vi "Begin.vi"() -> (0 "error out":errorcluster)   [LabVIEW 2014]
doc: "Called before other user functions, this VI is expected to open initial I/O refnums, load in file data, and do all program initialization. Notice that the <B>error out</B> terminal is simply used for data flow. Wiring it to other structures or subVIs ensures that this VI runs first."
uses:
  <vilib>/Rock Robotics/WPI/DriverStation/WPI_DriverStationRobotMode2.ctl
  <vilib>/Rock Robotics/WPI/Relay/WPI_RelayDirection.ctl
  <vilib>/Rock Robotics/SystemInterfaces/Typedef/FPGA_TypedefDigitalModule.ctl
  <vilib>/Rock Robotics/WPI/SafetyOutput/WPI_SafetyOutputConfigMenu.ctl
  <vilib>/Rock Robotics/WPI/Joystick/WPI_JoystickDeviceEnum.ctl
  <vilib>/Rock Robotics/SystemInterfaces/DIO/FPGA_DIOChannel.ctl
  <vilib>/Rock Robotics/WPI/Encoder/WPI_EncoderType.ctl
  <vilib>/Rock Robotics/SystemInterfaces/AI/FPGA_AIGyroChannel.ctl
  <vilib>/Rock Robotics/SystemInterfaces/Typedef/FPGA_TypedefAnalogModuleForGyro.ctl
  <vilib>/Rock Robotics/SystemInterfaces/AI/FPGA_AIChannel.ctl
  <vilib>/Rock Robotics/SystemInterfaces/DIO/FPGA_DIORelayChannel.ctl
  <vilib>/Rock Robotics/WPI/CAN/Jaguar/SubVIs/WPI_CANJaguar_ControlMode.ctl
  Robot Global Data.vi
  <vilib>/Rock Robotics/WPI/RobotDrive/WPI_RobotDriveOpen4MotorWithCANJaguar.vi
  <vilib>/Rock Robotics/WPI/Counter/WPI_CounterDigitalInputToDigitalSource.vi
  <vilib>/Rock Robotics/WPI/Ultrasonic/WPI_SonarMB1010AnalogOpen.vi
  <vilib>/Rock Robotics/WPI/Ultrasonic/WPI_SonarMB1010AnalogRefNum Registry Set.vi
  <vilib>/Rock Robotics/WPI/MotorControl/WPI_MotorControlOpenCANJaguar.vi
  <vilib>/Rock Robotics/WPI/Camera/WPI_CameraFrameRate.ctl
  <vilib>/Rock Robotics/WPI/Camera/WPI_CameraWhite Balance Values.ctl
  <vilib>/Rock Robotics/WPI/Camera/WPI_CameraExposure Values.ctl
  <vilib>/Rock Robotics/WPI/Camera/WPI_CameraImageSize.ctl
  <vilib>/Rock Robotics/WPI/Camera/WPI_CameraExposure Priority Values.ctl
  <vilib>/Rock Robotics/SystemInterfaces/Typedef/FPGA_TypedefAnalogModule.ctl
panel:
  # "Launch Angle Position PID"
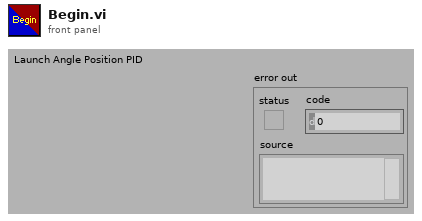
[diagram p1: front panel]
types:
  T1 = typedef "WPI_SafetyOutputConfigMenu.ctl" = enum16{"Enable", "Disable"}
  T2 = typedef "FPGA_TypedefDigitalModule.ctl" = enum16{"Controller 1"}
  T3 = typedef "WPI_RelayDirection.ctl" = enum16{"Both directions", "Forward only", "Reverse only"}
  T4 = typedef "WPI_DriverStationRobotMode2.ctl" = enum16{"Autonomous Disabled", "Autonomous Enabled", "Teleop Disabled", "Teleop Enabled", "Disconnected", "Finish", "Test Disabled", "Test Enabled"}
  T5 = typedef "WPI_JoystickDeviceEnum.ctl" = enum16{"USB 0", "USB 1", "USB 2", "USB 3", "USB 4", "USB 5"}
  T6 = typedef "WPI_CameraExposure Priority Values.ctl" = enum16{"None", "Prioritize frame rate", "Prioritize image quality"}
  T7 = typedef "WPI_CameraImageSize.ctl" = enum16{"640x480", "320x240", "160x120", "Custom"}
  T8 = typedef "WPI_CameraExposure Values.ctl" = enum16{"Auto", "Flicker-free 50 Hz", "Flicker-free 60 Hz", "Hold current", "Custom"}
  T9 = typedef "WPI_CameraWhite Balance Values.ctl" = enum16{"Auto", "Fixed indoor", "Fixed outdoor 1", "Fixed outdoor 2", "Fixed fluorescent 1", "Fixed fluorescent 2", "Hold current", "Custom"}
  T10 = typedef "WPI_CameraFrameRate.ctl" = u32
  T11 = typedef "FPGA_DIOChannel.ctl" = enum8{"DIO 0", "DIO 1", "DIO 2", "DIO 3", "DIO 4", "DIO 5", "DIO 6", "DIO 7", "DIO 8", "DIO 9", "DIO MXP 0", "DIO MXP 1", "DIO MXP 2", "DIO MXP 3", "DIO MXP 4", "DIO MXP 5", "DIO MXP 6", "DIO MXP 7", "DIO MXP 8", "DIO MXP 9", "DIO MXP 10", "DIO MXP 11", "DIO MXP 12", "DIO MXP 13", "DIO MXP 14", "DIO MXP 15", "Invalid"}
  T12 = typedef "FPGA_TypedefAnalogModuleForGyro.ctl" = enum16{"Controller 1"}
  T13 = typedef "FPGA_AIGyroChannel.ctl" = enum8{"AI 0", "AI 1", "Invalid"}
  T14 = typedef "FPGA_TypedefAnalogModule.ctl" = enum16{"Controller 1"}
  T15 = typedef "FPGA_AIChannel.ctl" = enum8{"AI 0", "AI 1", "AI 2", "AI 3", "AI MXP 0", "AI MXP 1", "AI MXP 2", "AI MXP 3", "Invalid"}
  T16 = typedef "FPGA_DIORelayChannel.ctl" = enum8{"Relay 0", "Relay 1", "Relay 2", "Relay 3", "Invalid"}
  T17 = typedef "WPI_CANJaguar_ControlMode.ctl" = enum8{"Percent VBus", "Current", "Speed", "Position", "Voltage"}
  T18 = typedef "WPI_JoystickDevRef.ctl" = cluster{"Device":T5}
  T19 = typedef "WPI_CameraDevRef.ctl" = cluster{"Camera Address":string, "CameraStatus":errorcluster}
  T20 = typedef "WPI_RobotDriveDevRef.ctl" = cluster{"DevStatus":errorcluster, "Motors[]":T21[], "Square Inputs":bool, "Max Output":dbl}
  T21 = typedef "WPI_MotorControlDeviceRef.ctl" = cluster{"DeviceStatus":errorcluster, "Type":enum16{"PWM", "CAN"}, "PWM":cluster{"Controller":T2, "PWM Channel":T22, "DeadBand":T23}, "CAN":cluster{"Device Number":u8, "Control Mode":T17, "Semaphore":T24, "Max Vout":dbl}, "Invert":bool, "TransformRef":T25, "InvTransformRef":T25}
  T22 = typedef "FPGA_DIOPWMChannel.ctl" = enum8{"PWM 0", "PWM 1", "PWM 2", "PWM 3", "PWM 4", "PWM 5", "PWM 6", "PWM 7", "PWM 8", "PWM 9", "PWM MXP 0", "PWM MXP 1", "PWM MXP 2", "PWM MXP 3", "PWM MXP 4", "PWM MXP 5", "PWM MXP 6", "PWM MXP 7", "PWM MXP 8", "PWM MXP 9", "Invalid"}
  T23 = typedef "WPI_PWMDeadband.ctl" = cluster{"Name":string, "maxPositivePwm":i32, "minPositivePwm":i32, "centerPwm":i32, "maxNegativePwm":i32, "minNegativePwm":i32, "angularRange":u16}
  T24 = typedef "Semaphore RefNum" = refnum<k1>
  T25 = typedef "WPI_PWMTransform_ConPane.ctl" = refnum<vi>
  T26 = typedef "WPI_EncoderType.ctl" = enum16{"1x", "2x", "4x"}
  T27 = typedef "WPI_DigitalInputDevRef.ctl" = cluster{"DevStatus":errorcluster, "DIO Channel":T11, "Controller":T2}
  T28 = typedef "FPGA_CounterEncoderSourceConvertionLVSourceType.ctl" = cluster{"DevStatus":errorcluster, "AnalogTriggerMode?":bool, "DigitalMode":cluster{"Controller":T2, "DIO Channel":T29}, "AnalogTriggerMode":cluster{"AnalogTriggerIndex":T30, "OutputType":T31}}
  T29 = typedef "FPGA_DIODigitalSourceChannel.ctl" = enum8{"DIO 0", "DIO 1", "DIO 2", "DIO 3", "DIO 4", "DIO 5", "DIO 6", "DIO 7", "DIO 8", "DIO 9", "DIO MXP 0", "DIO MXP 1", "DIO MXP 2", "DIO MXP 3", "DIO MXP 4", "DIO MXP 5", "DIO MXP 6", "DIO MXP 7", "DIO MXP 8", "DIO MXP 9", "DIO MXP 10", "DIO MXP 11", "DIO MXP 12", "DIO MXP 13", "DIO MXP 14", "DIO MXP 15", "Disabled"}
  T30 = typedef "FPGA_AnalogTriggerIndex.ctl" = enum8{"Trig 0", "Trig 1", "Trig 2", "Trig 3", "Trig 4", "Trig 5", "Trig 6", "Trig 7", "Invalid"}
  T31 = typedef "FPGA_AnalogTriggerOutType.ctl" = enum16{"InWindow", "TriggerState", "Rising", "Falling"}
  T32 = typedef "WPI_EncoderDevRef.ctl" = cluster{"DevStatus":errorcluster, "EncoderIndex":T33, "CounterIndex":T34, "DistancePerCount":dbl, "Decoding Type":T26}
  T33 = typedef "FPGA_EncoderIdx.ctl" = enum8{"Enc 0", "Enc 1", "Enc 2", "Enc 3", "Invalid"}
  T34 = typedef "FPGA_CounterCtrSystemIndex.ctl" = enum8{"Ctr 0", "Ctr 1", "Ctr 2", "Ctr 3", "Ctr 4", "Ctr 5", "Ctr 6", "Ctr 7", "Invalid"}
  T35 = typedef "WPI_GyroDevRef.ctl" = cluster{"DevStatus":errorcluster, "Analog Module":T14, "Analog Channel":T15, "Offset":dbl, "Gain (VoltsPerDegree/Second)":dbl}
  T36 = typedef "WPI_AnalogChannelDevRef.ctl" = cluster{"DevStatus":errorcluster, "Controller":T14, "Analog Channel":T15}
  T37 = typedef "WPI_SonarMB1010AnalogDeviceRef.ctl" = cluster{"AIDeviceRef":T36, "Scaling factor (V/in)":dbl, "Average Bits":u8}
  T38 = typedef "WPI_RelayDevRef.ctl" = cluster{"DevStatus":errorcluster, "Relay Channel":T16, "Controller":T2, "Relay Direction":T3}
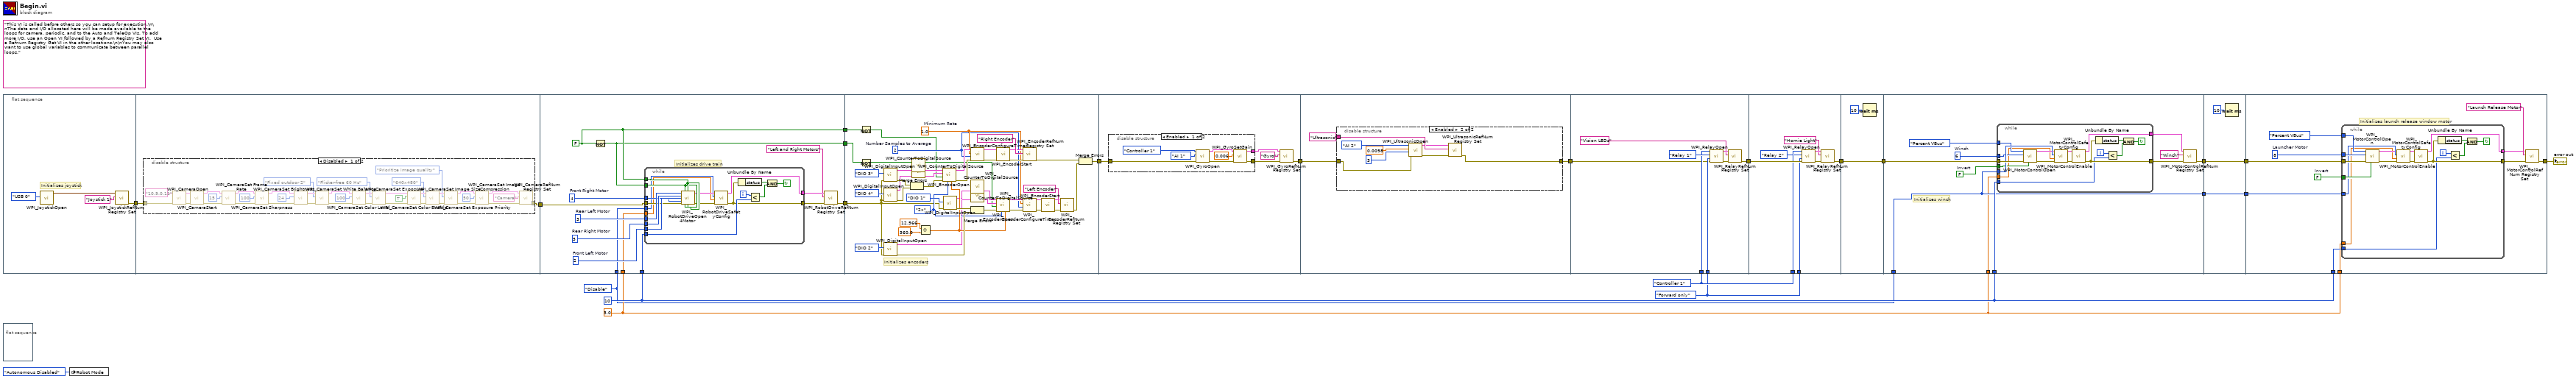
[diagram p0: block diagram]
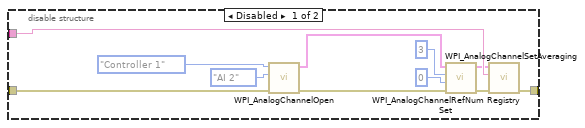
[diagram p4: hidden frame]
diagram:
  w10 = WPI_SafetyOutputConfigMenu."Disable" ("mode")
  w11 = 3.0 ("timeout (s)")
  w7 = FPGA_TypedefDigitalModule."Controller 1" ("Digital Module (Module 1)")
  w6 = WPI_RelayDirection."Forward only" ("Relay Direction")
  w13 = 10 ("y")
  (unwired) "This VI is called before others so you can setup for execution.\n\nThe data and I/O allocated here will be made available to the loops for camera, periodic, and to the Auto and TeleOp VIs. To add more I/O, use an Open VI followed by a Refnum Registry Set VI.  Use a Refnum Registry Get VI in the other locations.\n\nYou may also want to use global variables to communicate between parallel loops."
  n1 = flat-sequence {
    tunnel: [w23] -> w5
    tunnel: w5 -> [w28]
    tunnel: [w27] -> w1
    tunnel: [w73] -> w22
    tunnel: [w72] -> w21
    tunnel: [w71] -> w20
    tunnel: w13 -> [w70]
    tunnel: w11 -> [w69]
    tunnel: w10 -> [w68]
    tunnel: w1 -> [w67]
    tunnel: w20 -> [w104]
    tunnel: w21 -> [w103]
    tunnel: w22 -> [w102]
    tunnel: [w99] -> w12
    tunnel: [w145] -> w8
    tunnel: w12 -> [w149]
    tunnel: w8 -> [w160]
    tunnel: [w158] -> w2
    tunnel: w6 -> [w183]
    tunnel: w7 -> [w182]
    tunnel: [w181] -> w9
    tunnel: w2 -> [w180]
    tunnel: w9 -> [w192]
    tunnel: w6 -> [w191]
    tunnel: w7 -> [w190]
    tunnel: [w188] -> w4
    tunnel: [w196] -> w14
    tunnel: w4 -> [w196]
    tunnel: [w207] -> w18
    tunnel: [w199] -> w16
    tunnel: w13 -> [w204]
    tunnel: w14 -> [w200]
    tunnel: w10 -> [w199]
    tunnel: w11 -> [w198]
    tunnel: w18 -> [w228]
    tunnel: [w228] -> w17
    tunnel: w16 -> [w227]
    tunnel: [w227] -> w15
    tunnel: w17 -> [w235]
    tunnel: w15 -> [w234]
    tunnel: w13 -> [w231]
    tunnel: w11 -> [w230]
    tunnel: [w229] -> w3
    frame #0 {
      # "Initializes joystick"
      n2 = call <vilib>:"WPI_JoystickOpen.vi"("JoystickDevice"=WPI_JoystickDeviceEnum."USB 0") -> ("JoystickDevRef"=w25:T18)  [unwired: 10 in]
      n3 = call <vilib>:"WPI_JoystickRefNum Registry Set.vi"("refnum name"="Joystick 1", "JoystickDevRef"=w25) -> ("error out"=w23:errorcluster)  [unwired: 8 in, 1 out]
    }
    frame #1 {
      n4 = disable-structure shown="Disabled" {
        disable-tunnel: w28 -> [w66 _]
        disable-tunnel: [w29 _] -> w27
        frame Disabled {
          n5 = call <vilib>:"WPI_CameraOpen.vi"("error in (no error)"=w66, "Camera Address"="10.9.0.11") -> ("error out"=w65:errorcluster, "CameraDevRef"=w63:T19)  [unwired: 8 in]
          n6 = call <vilib>:"WPI_CameraStart.vi"("error in (no error)"=w65, "CameraDevRef"=w63) -> ("error out"=w60:errorcluster, "CameraDevRef Out"=w61:T19)  [unwired: 8 in]
          n7 = call <vilib>:"WPI_CameraSet Frame Rate.vi"("error in (no error)"=w60, "Frame Rate (fps)"=T10 15, "CameraDevRef"=w61) -> ("error out"=w58:errorcluster, "CameraDevRef Out"=w59:T19)  [unwired: 7 in]
          n8 = call <vilib>:"WPI_CameraSet Sharpness.vi"("error in (no error)"=w58, "Sharpness"=100, "CameraDevRef"=w59) -> ("error out"=w56:errorcluster, "CameraDevRef Out"=w57:T19)  [unwired: 7 in]
          n9 = call <vilib>:"WPI_CameraSet Brightness.vi"("error in (no error)"=w56, "Brightness"=24, "CameraDevRef"=w57) -> ("error out"=w54:errorcluster, "CameraDevRef Out"=w55:T19)  [unwired: 7 in]
          n10 = call <vilib>:"WPI_CameraSet White Balance.vi"("error in (no error)"=w54, "White Balance"=WPI_CameraWhite_Balance_Values."Fixed outdoor 2", "CameraDevRef"=w55) -> ("error out"=w52:errorcluster, "CameraDevRef Out"=w53:T19)  [unwired: 7 in]
          n11 = call <vilib>:"WPI_CameraSet Color Level.vi"("error in (no error)"=w52, "Color Level"=100, "CameraDevRef"=w53) -> ("error out"=w51:errorcluster, "CameraDevRef Out"=w50:T19)  [unwired: 7 in]
          n12 = call <vilib>:"WPI_CameraSet Exposure.vi"("error in (no error)"=w51, "Exposure"=WPI_CameraExposure_Values."Flicker-free 60 Hz", "CameraDevRef"=w50) -> ("error out"=w49:errorcluster, "CameraDevRef Out"=w48:T19)  [unwired: 7 in]
          n13 = call <vilib>:"WPI_CameraSet Color Enable.vi"("error in (no error)"=w49, "Color Enabled"=TRUE, "CameraDevRef"=w48) -> ("error out"=w46:errorcluster, "CameraDevRef Out"=w47:T19)  [unwired: 7 in]
          n14 = call <vilib>:"WPI_CameraSet Image Size.vi"("error in (no error)"=w46, "Image Size"=WPI_CameraImageSize."640x480", "CameraDevRef"=w47) -> ("error out"=w44:errorcluster, "CameraDevRef Out"=w45:T19)  [unwired: 7 in]
          n15 = call <vilib>:"WPI_CameraSet Exposure Priority.vi"("error in (no error)"=w44, "Exposure Priority"=WPI_CameraExposure_Priority_Values."Prioritize image quality", "CameraDevRef"=w45) -> ("error out"=w43:errorcluster, "CameraDevRef Out"=w42:T19)  [unwired: 7 in]
          n16 = call <vilib>:"WPI_CameraSet Image Compression.vi"("error in (no error)"=w43, "Compression"=50, "CameraDevRef"=w42) -> ("error out"=w40:errorcluster, "CameraDevRef Out"=w41:T19)  [unwired: 7 in]
          n17 = call <vilib>:"WPI_CameraRefNum Registry Set.vi"("error in (no error)"=w40, "refnum name"="Camera", "CameraDevRef"=w41) -> ("error out"=w29:errorcluster)  [unwired: 7 in, 1 out]
        }
        frame Enabled {
        }
      }
    }
    frame #2 {
      w72 = FALSE ("Rear Left Motor Inverted")
      w74 = u8 4  # Front Right Motor
      w75 = u8 2  # Front Left Motor
      w76 = u8 5  # Rear Right Motor
      w77 = u8 3  # Rear Left Motor
      # "Initializes drive train"
      n18 = Not(x=w72) -> (.not. x?=w71:bool)
      n19 = while {
        tunnel: [w85] -> w80
        tunnel: [w86] -> w79
        tunnel: w77 -> [w98]
        tunnel: w76 -> [w97]
        tunnel: w75 -> [w96]
        tunnel: w74 -> [w95]
        tunnel: w67 -> [w94]
        tunnel: w72 -> [w93]
        tunnel: w71 -> [w92]
        tunnel: w70 -> [w88]
        tunnel: w68 -> [w82]
        tunnel: w69 -> [w81]
        i -> [w89]
        stop <- w91 continue-if-true
        n20 = call-poly <vilib>:"WPI_RobotDriveOpen4Motor.vi"("Rear Left Motor"=w98, "Rear Left Motor Inverted"=w92, "Rear Right Motor Inverted"=w93, "Rear Right Motor"=w97, "Front Left Motor"=w96, "Front Right Motor"=w95, "error in (no error)"=w94, "Front Left Motor Inverted"=w92, "Front Right Motor Inverted"=w93) -> ("RobotDriveDevRef"=w84:T20, "error out"=w83:errorcluster)  [unwired: 5 in]
        n21 = call <vilib>:"WPI_RobotDriveSafetyConfig.vi"("error in (no error)"=w83, "timeout (s)"=w81, "mode"=w82, "RobotDriveDevRef"=w84) -> ("error out"=w85:errorcluster, "RobotDriveDevRef"=w86:T20)  [unwired: 6 in]
        n22 = Unbundle By Name(w85) -> ("status"=w90:bool)
        n23 = Less?(x=w89, y=w88) -> (x < y?=w87:bool)
        n24 = And(x=w90, y=w87) -> (x .and. y?=w91:bool)
      }
      n25 = call <vilib>:"WPI_RobotDriveRefNum Registry Set.vi"("error in (no error)"=w80, "refnum name"="Left and Right Motors", "RobotDriveDevRef"=w79) -> ("error out"=w73:errorcluster)  [unwired: 7 in, 1 out]
    }
    frame #3 {
      w112 = u8 2  # Number Samples to Average
      w113 = 1.0  # Minimum Rate
      w122 = WPI_EncoderType."2x" ("Decoding Type")
      # "Initializes encoders"
      n26 = Not(x=w103) -> (.not. x?=w106:bool)
      n27 = Not(x=w104) -> (.not. x?=w107:bool)
      n28 = call <vilib>:"WPI_DigitalInputOpen.vi"("error in (no error)"=w102, "DIO Channel"=FPGA_DIOChannel."DIO 3") -> ("error out"=w143:errorcluster, "DigitalInputDevRef"=w111:T27)  [unwired: 8 in]
      n29 = call <vilib>:"WPI_DigitalInputOpen.vi"("error in (no error)"=w102, "DIO Channel"=FPGA_DIOChannel."DIO 4") -> ("error out"=w142:errorcluster, "DigitalInputDevRef"=w110:T27)  [unwired: 8 in]
      n30 = call <vilib>:"WPI_DigitalInputOpen.vi"("error in (no error)"=w102, "DIO Channel"=FPGA_DIOChannel."DIO 2") -> ("error out"=w137:errorcluster, "DigitalInputDevRef"=w109:T27)  [unwired: 8 in]
      n31 = Merge Errors(w143, w142) -> (w141:errorcluster)
      n32 = call-poly <vilib>:"WPI_CounterToDigitalSource.vi"("DigitalInputDevRef"=w111) -> ("Digital Source"=w144:T28)  [unwired: 6 in]
      n33 = call-poly <vilib>:"WPI_CounterToDigitalSource.vi"("DigitalInputDevRef"=w110) -> ("Digital Source"=w140:T28)  [unwired: 6 in]
      n34 = Divide(x=12.566, y=360.0) -> (x/y=w127:dbl)
      n35 = call <vilib>:"WPI_EncoderOpen.vi"("DistancePerCount"=w127, "Decoding Type"=w122, "error in (no error)"=w141, "Invert Direction (False)"=w106, "BSource"=w140, "ASource"=w144) -> ("error out"=w114:errorcluster, "EncoderDevRef"=w117:T32)  [unwired: 4 in]
      n36 = call <vilib>:"WPI_DigitalInputOpen.vi"("error in (no error)"=w102, "DIO Channel"=FPGA_DIOChannel."DIO 1") -> ("error out"=w138:errorcluster, "DigitalInputDevRef"=w108:T27)  [unwired: 8 in]
      n37 = call <vilib>:"WPI_EncoderConfigureTimer.vi"("error in (no error)"=w114, "Number Samples to Average"=w112, "Minimum Rate"=w113, "EncoderDevRef"=w117) -> ("error out"=w115:errorcluster, "EncoderDevRef"=w116:T32)  [unwired: 6 in]
      n38 = call-poly <vilib>:"WPI_CounterToDigitalSource.vi"("DigitalInputDevRef"=w108) -> ("Digital Source"=w139:T28)  [unwired: 6 in]
      n39 = call-poly <vilib>:"WPI_CounterToDigitalSource.vi"("DigitalInputDevRef"=w109) -> ("Digital Source"=w135:T28)  [unwired: 6 in]
      n40 = Merge Errors(w138, w137) -> (w136:errorcluster)
      n41 = call <vilib>:"WPI_EncoderOpen.vi"("DistancePerCount"=w127, "Decoding Type"=w122, "error in (no error)"=w136, "Invert Direction (False)"=w107, "BSource"=w135, "ASource"=w139) -> ("error out"=w120:errorcluster, "EncoderDevRef"=w121:T32)  [unwired: 4 in]
      n42 = call <vilib>:"WPI_EncoderStart.vi"("error in (no error)"=w115, "EncoderDevRef"=w116) -> ("error out"=w123:errorcluster, "EncoderDevRef"=w124:T32)  [unwired: 8 in]
      n43 = call <vilib>:"WPI_EncoderRefNum Registry Set.vi"("error in (no error)"=w123, "refnum name"="Right Encoder", "EncoderDevRef"=w124) -> ("error out"=w101:errorcluster)  [unwired: 7 in, 1 out]
      n44 = call <vilib>:"WPI_EncoderConfigureTimer.vi"("error in (no error)"=w120, "Number Samples to Average"=w112, "Minimum Rate"=w113, "EncoderDevRef"=w121) -> ("error out"=w118:errorcluster, "EncoderDevRef"=w119:T32)  [unwired: 6 in]
      n45 = call <vilib>:"WPI_EncoderStart.vi"("error in (no error)"=w118, "EncoderDevRef"=w119) -> ("error out"=w125:errorcluster, "EncoderDevRef"=w126:T32)  [unwired: 8 in]
      n46 = call <vilib>:"WPI_EncoderRefNum Registry Set.vi"("error in (no error)"=w125, "refnum name"="Left Encoder", "EncoderDevRef"=w126) -> ("error out"=w100:errorcluster)  [unwired: 7 in, 1 out]
      n47 = Merge Errors(w101, w100) -> (w99:errorcluster)
    }
    frame #4 {
      n48 = disable-structure shown="Enabled" {
        disable-tunnel: w149 -> [w157 _]
        disable-tunnel: [w151 _] -> w146
        disable-tunnel: [w150 _] -> w148
        frame Enabled {
          n49 = call <vilib>:"WPI_GyroOpen.vi"("error in (no error)"=w157, "Analog Channel"=FPGA_AIGyroChannel."AI 1", "Controller"=FPGA_TypedefAnalogModuleForGyro."Controller 1" ("Analog Module (Module 1)")) -> ("error out"=w154:errorcluster, "GyroDevRef"=w153:T35)  [unwired: 6 in, 1 out]
          n50 = call <vilib>:"WPI_GyroSetGain.vi"("error in (no error)"=w154, "Gain (VoltsPerDegree/Second)"=0.006, "GyroDevRef"=w153) -> ("error out"=w150:errorcluster, "GyroDevRef"=w151:T35)  [unwired: 7 in]
        }
        frame Disabled {
        }
      }
      n51 = call <vilib>:"WPI_GyroRefNum Registry Set.vi"("error in (no error)"=w148, "refnum name"="Gyro", "GyroDevRef"=w146) -> ("error out"=w145:errorcluster)  [unwired: 7 in, 1 out]
    }
    frame #5 {
      n52 = disable-structure shown="Enabled" {
        disable-tunnel: w160 -> [w171 w179]
        disable-tunnel: [w164 w175] -> w158
        disable-tunnel: "Ultrasonic" ("refnum name") -> [w166 w173]
        frame Disabled {
          n53 = call <vilib>:"WPI_AnalogChannelOpen.vi"("error in (no error)"=w171, "Analog Channel"=FPGA_AIChannel."AI 2", "Controller"=FPGA_TypedefAnalogModule."Controller 1" ("Analog Module (Module 1)")) -> ("error out"=w161:errorcluster, "AIDeviceRef"=w170:T36)  [unwired: 7 in]
          n54 = call <vilib>:"WPI_AnalogChannelSetAveraging.vi"("error in (no error)"=w161, "OversampleBits"=u8 0, "AverageBits"=u8 3, "AIDeviceRef"=w170) -> ("error out"=w163:errorcluster, "AIDeviceRef"=w165:T36)  [unwired: 6 in]
          n55 = call <vilib>:"WPI_AnalogChannelRefNum Registry Set.vi"("error in (no error)"=w163, "refnum name"=w166, "AIDeviceRef"=w165) -> ("error out"=w164:errorcluster)  [unwired: 7 in, 1 out]
        }
        frame Enabled {
          n56 = call-poly <vilib>:"WPI_UltrasonicOpen.vi"("error in"=w179, "Average Bits"=u8 3, "Scaling factor (V/in)"=0.0098, "Analog Channel"=FPGA_AIChannel."AI 2") -> ("error out"=w174:errorcluster, "SonarMB1010AnalogDevRef"=w172:T37)  [unwired: 6 in]
          n57 = call-poly <vilib>:"WPI_UltrasonicRefNum Registry Set.vi"("error in (no error)"=w174, "refnum name"=w173, "SonarMB1010AnalogDevRef"=w172) -> ("error out"=w175:errorcluster)  [unwired: 7 in, 1 out]
        }
      }
    }
    frame #6 {
      n58 = call <vilib>:"WPI_RelayOpen.vi"("error in (no error)"=w180, "Relay Direction"=w183, "Relay Channel"=FPGA_DIORelayChannel."Relay 1", "Controller"=w182) -> ("error out"=w187:errorcluster, "RelayDevRef"=w186:T38)  [unwired: 6 in]
      n59 = call <vilib>:"WPI_RelayRefNum Registry Set.vi"("error in (no error)"=w187, "refnum name"="Vision LEDs", "RelayDevRef"=w186) -> ("error out"=w181:errorcluster)  [unwired: 7 in, 1 out]
    }
    frame #7 {
      n60 = call <vilib>:"WPI_RelayOpen.vi"("error in (no error)"=w192, "Relay Direction"=w191, "Relay Channel"=FPGA_DIORelayChannel."Relay 2", "Controller"=w190) -> ("error out"=w195:errorcluster, "RelayDevRef"=w194:T38)  [unwired: 6 in]
      n61 = call <vilib>:"WPI_RelayRefNum Registry Set.vi"("error in (no error)"=w195, "refnum name"="Homie Light", "RelayDevRef"=w194) -> ("error out"=w188:errorcluster)  [unwired: 7 in, 1 out]
    }
    frame #8 {
      n62 = Wait (ms)(milliseconds to wait=u32 10) -> ()  [unwired: 1 out]
    }
    frame #9 {
      w201 = FALSE  # Invert
      w202 = u8 6  # Winch
      # "Initializes winch"
      n63 = while {
        tunnel: w200 -> [w223]
        tunnel: w199 -> [w222]
        tunnel: [w218] -> w206
        tunnel: [w219] -> w205
        tunnel: w204 -> [w216]
        tunnel: WPI_CANJaguar_ControlMode."Percent VBus" ("Control Mode") -> [w212]
        tunnel: w202 -> [w211]
        tunnel: w201 -> [w210]
        tunnel: w198 -> [w209]
        i -> [w217]
        stop <- w213 continue-if-true
        n64 = call-poly <vilib>:"WPI_MotorControlOpen.vi"("Invert"=w210, "error in (no error)"=w223, "Device Number"=w211, "Control Mode"=w212) -> ("error out"=w220:errorcluster, "MotorControlDeviceRef"=w221:T21)  [unwired: 6 in]
        n65 = call <vilib>:"WPI_MotorControlSafetyConfig.vi"("error in (no error)"=w220, "timeout (s)"=w209, "mode"=w222, "MotorControlDevRef"=w221) -> ("error out"=w225:errorcluster, "MotorControlDevRef"=w224:T21)  [unwired: 6 in]
        n66 = call <vilib>:"WPI_MotorControlEnable.vi"("error in (no error)"=w225, "CAN Jaguar Ref"=w224) -> ("error out"=w218:errorcluster, "CAN Jaguar Ref Out"=w219:T21)  [unwired: 8 in]
        n67 = Unbundle By Name(w218) -> ("status"=w214:bool)
        n68 = Less?(x=w217, y=w216) -> (x < y?=w215:bool)
        n69 = And(x=w214, y=w215) -> (x .and. y?=w213:bool)
      }
      n70 = call <vilib>:"WPI_MotorControlRefNum Registry Set.vi"("error in (no error)"=w206, "refnum name"="Winch", "MotorControlDevRef"=w205) -> ("error out"=w207:errorcluster)  [unwired: 7 in, 1 out]
    }
    frame #10 {
      n71 = Wait (ms)(milliseconds to wait=u32 10) -> ()  [unwired: 1 out]
    }
    frame #11 {
      w238 = u8 8  # Launcher Motor
      w239 = FALSE  # Invert
      # "Initializes launch release window motor"
      n72 = while {
        tunnel: w239 -> [w256]
        tunnel: w238 -> [w255]
        tunnel: WPI_CANJaguar_ControlMode."Percent VBus" ("Control Mode") -> [w254]
        tunnel: w235 -> [w251]
        tunnel: w234 -> [w250]
        tunnel: [w243] -> w233
        tunnel: [w247] -> w232
        tunnel: w231 -> [w241]
        tunnel: w230 -> [w240]
        i -> [w242]
        stop <- w246 continue-if-true
        n73 = call-poly <vilib>:"WPI_MotorControlOpen.vi"("Invert"=w256, "error in (no error)"=w251, "Device Number"=w255, "Control Mode"=w254) -> ("error out"=w248:errorcluster, "MotorControlDeviceRef"=w249:T21)  [unwired: 6 in]
        n74 = call <vilib>:"WPI_MotorControlSafetyConfig.vi"("error in (no error)"=w248, "timeout (s)"=w240, "mode"=w250, "MotorControlDevRef"=w249) -> ("error out"=w253:errorcluster, "MotorControlDevRef"=w252:T21)  [unwired: 6 in]
        n75 = call <vilib>:"WPI_MotorControlEnable.vi"("error in (no error)"=w253, "CAN Jaguar Ref"=w252) -> ("error out"=w243:errorcluster, "CAN Jaguar Ref Out"=w247:T21)  [unwired: 8 in]
        n76 = Unbundle By Name(w243) -> ("status"=w244:bool)
        n77 = Less?(x=w242, y=w241) -> (x < y?=w245:bool)
        n78 = And(x=w244, y=w245) -> (x .and. y?=w246:bool)
      }
      n79 = call <vilib>:"WPI_MotorControlRefNum Registry Set.vi"("error in (no error)"=w233, "refnum name"="Launch Release Motor", "MotorControlDevRef"=w232) -> ("error out"=w229:errorcluster)  [unwired: 7 in, 1 out]
    }
  }
  n80 = flat-sequence {
    frame #0 {
    }
  }
  n81 = global write "Robot Global Data.vi" "Robot Mode"(WPI_DriverStationRobotMode2."Autonomous Disabled" ("Robot Mode")) -> ()
  "error out" <- w3
